vi "harvestRegisters.vi"() -> ()   [LabVIEW 2020]
uses:
  <vilib>/Plasmionique/MB Master/MB_Master_TCP/MB_Master_TCP.lvclass
  Applications/National Instruments/LabVIEW 2020 64-bit/vi.lib/Plasmionique/MB Master/MB_Master/MB_Master.lvclass
  <vilib>/Plasmionique/MB Master/MB Master.lvlib
panel:
  out "Array":errorcluster[](array[cluster])
  in  "Slave ID (255)":u8=255
  in  "Port (502)":u16=502
  in  "Timeout (10000)":i32=1000
  in  "Stop":bool
  in  "startReg":u16=1600
  in  "IP Address":string="localhost"
  in  "nReg":i32=1600
  out "output":i32[][](array[numeric])
  out "error out":errorcluster
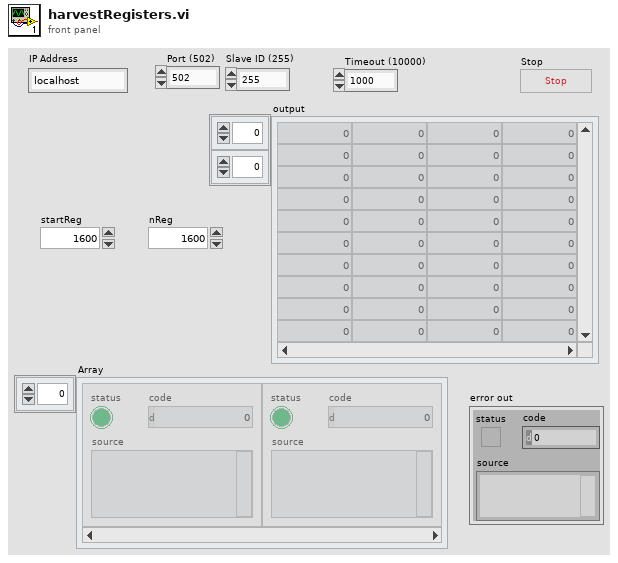
[diagram p1: front panel]
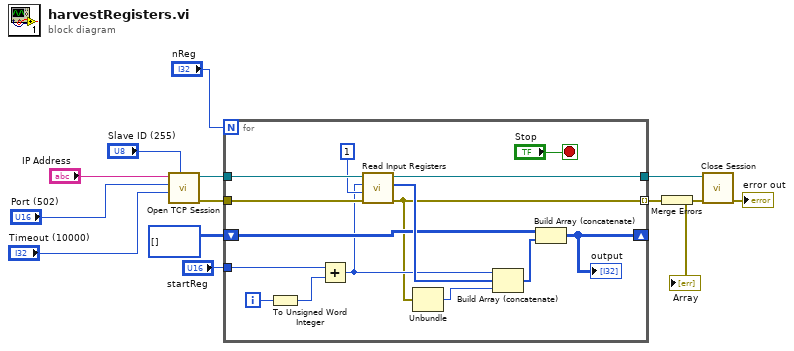
[diagram p0: block diagram]
diagram:
  n1 = call <vilib>:"Open TCP Session.vi"("Slave ID (255)"="Slave ID (255)", "Timeout (10000)"="Timeout (10000)", "Port (502)"="Port (502)", "IP Address"="IP Address") -> ("error out"=w10:errorcluster, "MB_TCP session"=w12:refnum<class "MB_Master_TCP.lvclass">)  [unwired: 6 in]
  n2 = for {
    N: "nReg" -> [_]
    tunnel: w12 -> [w28]
    tunnel: [w27] -> w11
    tunnel: w10 -> [w26]
    tunnel: [w17] -> w9 mode=indexing
    shift-right: [w20] -> _
    shift-left: u16[][] [] ("Array") -> [w22]
    tunnel: "startReg" -> [w18]
    i -> [w24]
    stop <- "Stop" stop-if-true
    n3 = To Unsigned Word Integer(number=w24) -> (unsigned 16bit integer=w15:u16)
    n4 = Add(x=w18, y=w15) -> (x+y=w19:u16)
    n5 = call <vilib>:"Read Input Registers.vi"("error in (no error)"=w26, "quantity"=u16 1, "starting address"=w19, "MB session in"=w28) -> ("error out"=w17:errorcluster, "Registers"=w23:u16[], "MB session out"=w27:refnum<class "MB_Master_TCP.lvclass">)  [unwired: 5 in]
    n6 = Unbundle(w17) -> ("code"=w14:i32)  [unwired: 2 out]
    n7 = Build Array (concatenate)(w19, w23, w14) -> (w21:i32[])
    n8 = Build Array (concatenate)(w22, w21) -> (w20:i32[][])
    "output" <- w20
  }
  "Array" <- w9
  n9 = Merge Errors(w9) -> (w8:errorcluster)
  n10 = call-dynamic "Close Session.vi"("error in (no error)"=w8, "MB TCP session"=w11) -> ("error out"=→"error out":errorcluster)  [unwired: 9 in]
